vi "getAllData.vi"(8 "error in (no error)":errorcluster) -> (0 "error out":errorcluster, 3 "AllData":T1)   [LabVIEW 2017, in "lowLevelController.lvlib"]
uses:
  lowLevelController.lvlib
  TypeDefs/allData.ctl
  TypeDefs/dataOut.ctl
  TypeDefs/dataIn.ctl
  SubVIs/FGVs/TypeDefs/DataFGVControl.ctl
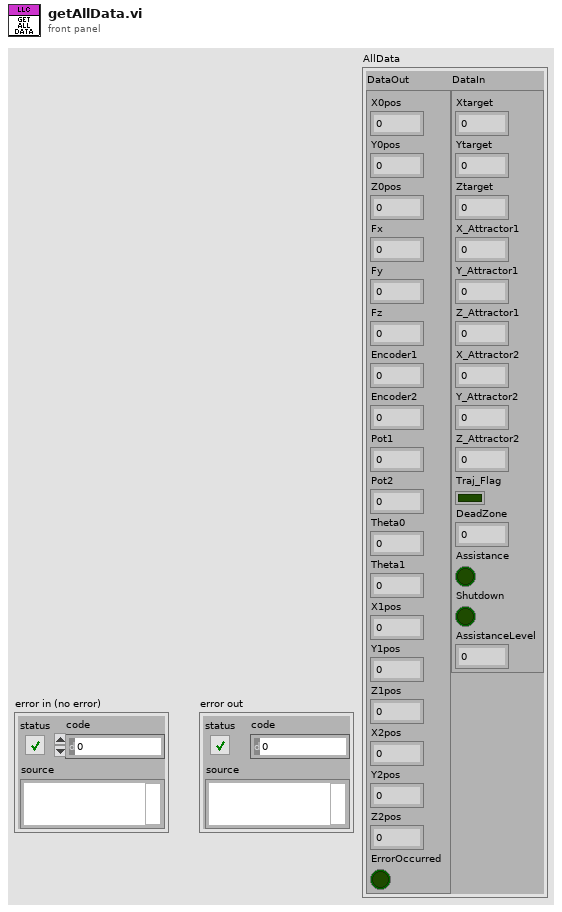
[diagram p1: front panel]
types:
  T1 = typedef "allData.ctl" = cluster{"DataOut":T2, "DataIn":T3}
  T2 = typedef "dataOut.ctl" = cluster{"X0pos":dbl, "Y0pos":dbl, "Z0pos":dbl, "Fx":dbl, "Fy":dbl, "Fz":dbl, "Encoder1":i32, "Encoder2":i32, "Pot1":dbl, "Pot2":dbl, "Theta0":dbl, "Theta1":dbl, "X1pos":dbl, "Y1pos":dbl, "Z1pos":dbl, "X2pos":dbl, "Y2pos":dbl, "Z2pos":dbl, "ErrorOccurred":bool}
  T3 = typedef "dataIn.ctl" = cluster{"Xtarget":dbl, "Ytarget":dbl, "Ztarget":dbl, "X_Attractor1":dbl, "Y_Attractor1":dbl, "Z_Attractor1":dbl, "X_Attractor2":dbl, "Y_Attractor2":dbl, "Z_Attractor2":dbl, "Traj_Flag":bool, "DeadZone":dbl, "Assistance":bool, "Shutdown":bool, "AssistanceLevel":dbl}
  T4 = typedef "DataFGVControl.ctl" = enum16{"init", "Set DataOut", "Get DataOut", "Set DataIn", "Get DataIn"}
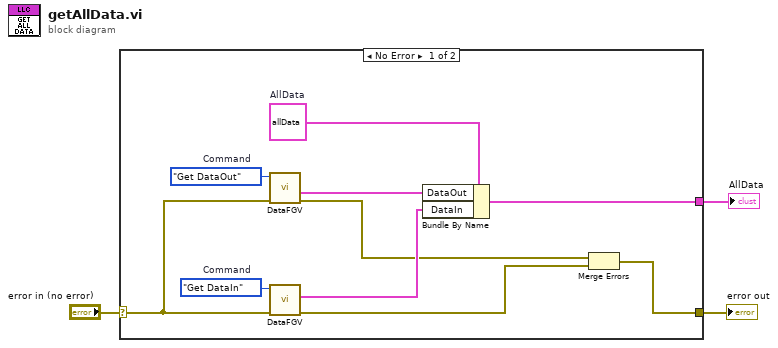
[diagram p0: block diagram]
diagram:
  n1 = case shown="No Error" "error in (no error)" {
    selector: "error in (no error)" -> [w4 w14]
    tunnel: [w8 _] -> w3
    tunnel: [w6 w14] -> w2
    frame No Error {
      w11 = T1 {"DataOut"={"X0pos"=0.0, "Y0pos"=0.0, "Z0pos"=0.0, "Fx"=0.0, "Fy"=0.0, "Fz"=0.0, "Encoder1"=0, "Encoder2"=0, "Pot1"=0.0, "Pot2"=0.0, "Theta0"=0.0, "Theta1"=0.0, "X1pos"=0.0, "Y1pos"=0.0, "Z1pos"=0.0, "X2pos"=0.0, "Y2pos"=0.0, "Z2pos"=0.0, "ErrorOccurred"=FALSE}, "DataIn"={"Xtarget"=0.0, "Ytarget"=0.0, "Ztarget"=0.0, "X_Attractor1"=0.0, "Y_Attractor1"=0.0, "Z_Attractor1"=0.0, "X_Attractor2"=0.0, "Y_Attractor2"=0.0, "Z_Attractor2"=0.0, "Traj_Flag"=FALSE, "DeadZone"=0.0, "Assistance"=FALSE, "Shutdown"=FALSE, "AssistanceLevel"=0.0}}  # AllData
      w12 = DataFGVControl."Get DataOut"  # Command
      w13 = DataFGVControl."Get DataIn"  # Command
      n2 = call "DataFGV.vi"("error in (no error)"=w4, "Command"=w12) -> ("error out"=w5:errorcluster, "DataOut"=w10:T2)  [unwired: 7 in, 1 out]
      n3 = call "DataFGV.vi"("error in (no error)"=w4, "Command"=w13) -> ("error out"=w7:errorcluster, "DataIn"=w9:T3)  [unwired: 7 in, 1 out]
      n4 = Bundle By Name(cluster=w11, "DataOut"=w10, "DataIn"=w9) -> (w8:T1)
      n5 = Merge Errors(w5, w7) -> (w6:errorcluster)
    }
    frame Error {
    }
  }
  "error out" <- w2
  "AllData" <- w3
